vi "RunMe (Test Launcher).vi"() -> ()   [LabVIEW 2020, in "Test Runner.JUnit.lvclass"]
uses:
  Test Runner.JUnit.lvclass
  C:/projects/caraya/src/classes/Test Runner/Test Runner.lvclass
  classes/Test Runner/Test Runner.lvclass
panel:
  out "error out":errorcluster
  # "RUN ME.\n\nThis VI runs the Tests related to JUnit Reporting."
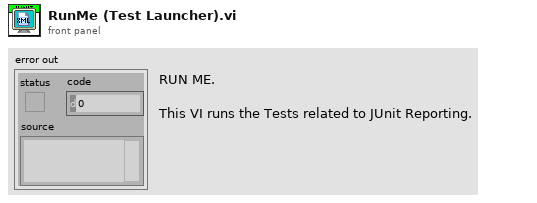
[diagram p1: front panel]
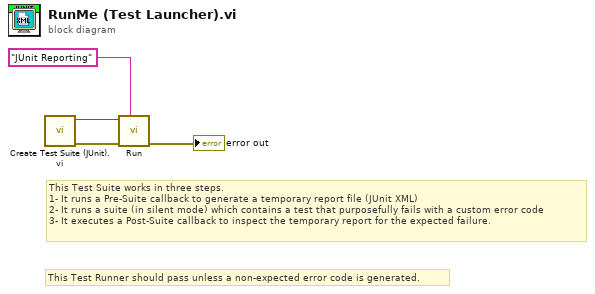
[diagram p0: block diagram]
diagram:
  # "This Test Runner should pass unless a non-expected error code is generated."
  # "This Test Suite works in three steps.\n1- It runs a Pre-Suite callback to generate a temporary report file (JUnit XML)\n2- It runs a suite (in silent mode) which contains a test that purposefully fails with a custom error code\n3- It executes a Post-Suite callback to inspect the temporary report for the expected failure."
  n1 = call "Create Test Suite (JUnit).vi.vi"() -> ("error out"=w3:errorcluster, "Test Runner.JUnit in"=w4:refnum<class "Test Runner.JUnit.lvclass">)  [unwired: 10 in]
  n2 = call "Run.vi"("Name"="JUnit Reporting", "error in (no error)"=w3, "Test Runner in"=w4) -> ("error out"=→"error out":errorcluster)  [unwired: 6 in, 2 out]
